vi "AlazarGetTriggerAddress.vi"(0 "Handle":u64, 1 "Record":u32, 5 "error in (no error)":errorcluster) -> (14 "Handle":u64, 15 "Trigger Address":u32, 16 "Timestamp High Part":u32, 17 "Timestamp Low Part":u32, 18 "Return Code":u32, 19 "error out":errorcluster)   [LabVIEW 2009]
doc: "Get the timestamp and trigger address of the trigger event in a record acquired to on-board memory."
uses:
  ATSApi.dll
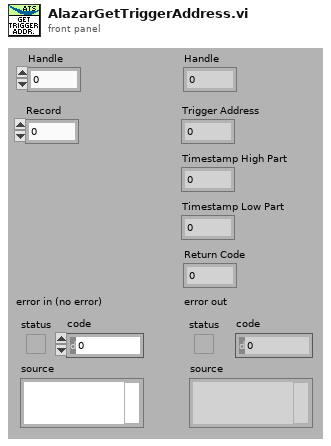
[diagram p1: front panel]
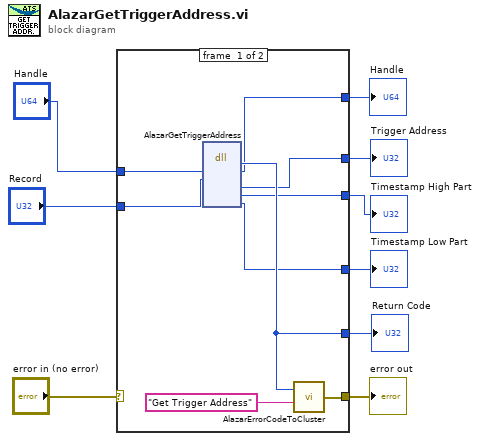
[diagram p0: block diagram]
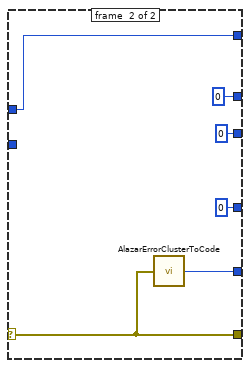
[diagram p2: hidden frame]
diagram:
  n1 = case shown="No Error" "error in (no error)" {
    selector: "error in (no error)" -> [_ w24]
    tunnel: [w15 w24] -> w8
    tunnel: "Handle" -> [w18 w22]
    tunnel: [w14 w22] -> w6
    tunnel: [w17 w23] -> w5
    tunnel: [w13 u32 0] -> w4
    tunnel: [w12 u32 0] -> w3
    tunnel: [w11 u32 0] -> w2
    tunnel: "Record" -> [w10 _]
    frame #0 {
      n2 = dll-call lib="ATSApi.dll" fn="AlazarGetTriggerAddress"("handle"=w18, "record"=w10) -> ("return type"=w17:u32, "handle"=w14:u64, "triggerAddress"=w11:u32, "timestampHighPart"=w12:u32, "timestampLowPart"=w13:u32)  [unwired: 7 in, 2 out]
      n3 = call "AlazarErrorCodeToCluster.vi"("Message"="Get Trigger Address", "Error Code"=w17) -> ("error out"=w15:errorcluster)
    }
    frame #1 {
      n4 = call "AlazarErrorClusterToCode.vi"("error in (no error)"=w24) -> ("Error Code"=w23:u32)
    }
  }
  "Handle" <- w6
  "error out" <- w8
  "Return Code" <- w5
  "Trigger Address" <- w2
  "Timestamp High Part" <- w3
  "Timestamp Low Part" <- w4
